vi "TestMode_Req_CMD_Abort.vi"(0 "Socket IP Address":string="192.168.1.100", 1 "Socket Port Number":u16=1600, 2 "Receipe Msg ID":i32=93, 3 "Receipe Message length":i32=36, 4 "Response ID":u8=94, 5 "error in (no error)":errorcluster, 6 "TestAmplitudeLoopC1":i32=500, 7 "TestFrequencyHigh":i32=500, 8 "TestAmplitudeLoopC2":i32=100, 9 "TestFrequencyLow":i32=450, 10 "TestPhaseLoopI":i32=300, 11 "TestAmplitude":i32=450, 12 "TestPhaseLoopCF":i32=500) -> (16 "Test Mode progress bar":string, 19 "error out":errorcluster)   [LabVIEW 2017]
panel:
  out "connection ID out":refnum<k5>
  # "Parameter Name                                        20KHz                                                                                                          \t40KHz\t\t\n\t                                        Default Value\t    Min Value\t       Max Value\t                                     Default Value         \tMin Value\t            Max Value\nTestAmplitudeLoopC1   100                         1                        20000                                               205                            1                             20000\nTestAmplitudeLoopC2   300                         1                        20000                                               370                            1                             20000\nTestPhaseLoopI               450                         50                      500                                                   60                             50                               500\nTestPhaseLoopCF           450                         50                       500                                                  200                           50                               500\nTestFrequencyHigh        20450                   Note                    Note                                                40900                      Note                           Note\nTestFrequencyLow          19450                   Note                   Note                                                38900                       Note                           Note\nTestAmplitude                 50                           10                       100                                                  50                             10                                100\n\nNote:  FreqLow and FreqHigh cannot cross and must remain within the band"
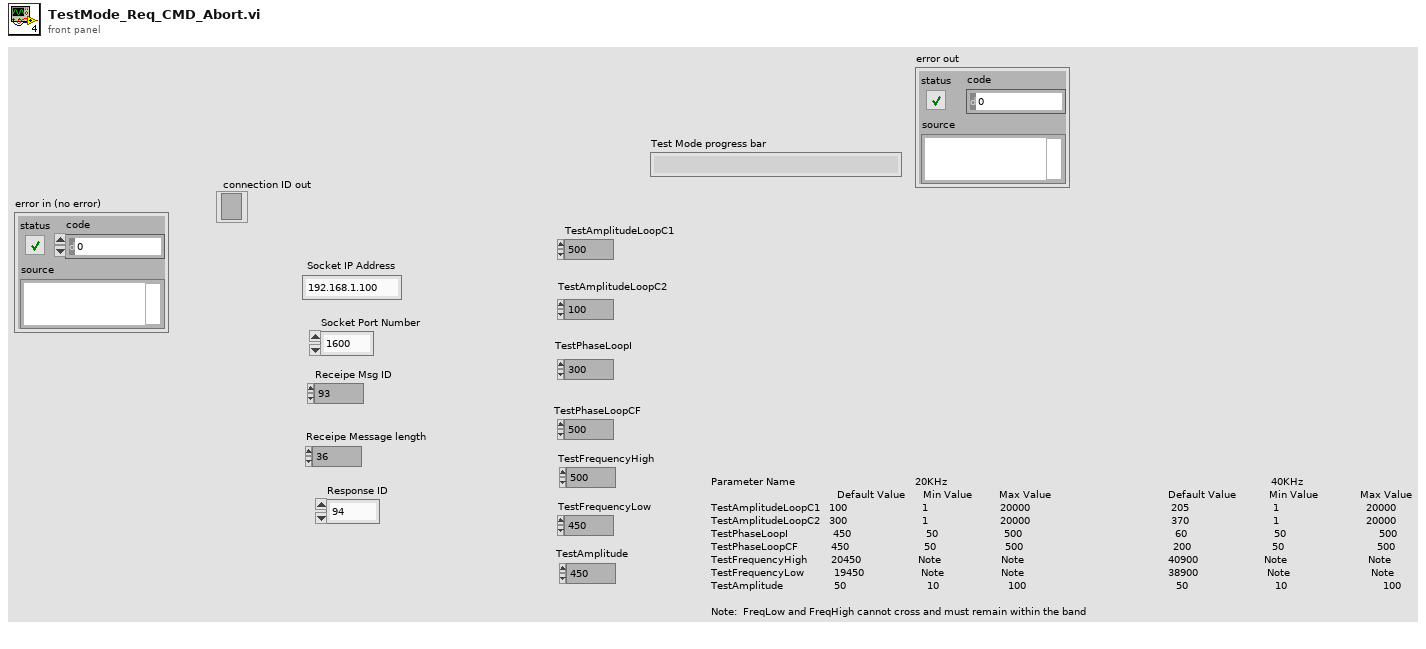
[diagram p1: front panel]
types:
  T1 = cluster{"Seek Request Message Length to DB ":i32, "Seek Request Message ID to DB":i32}
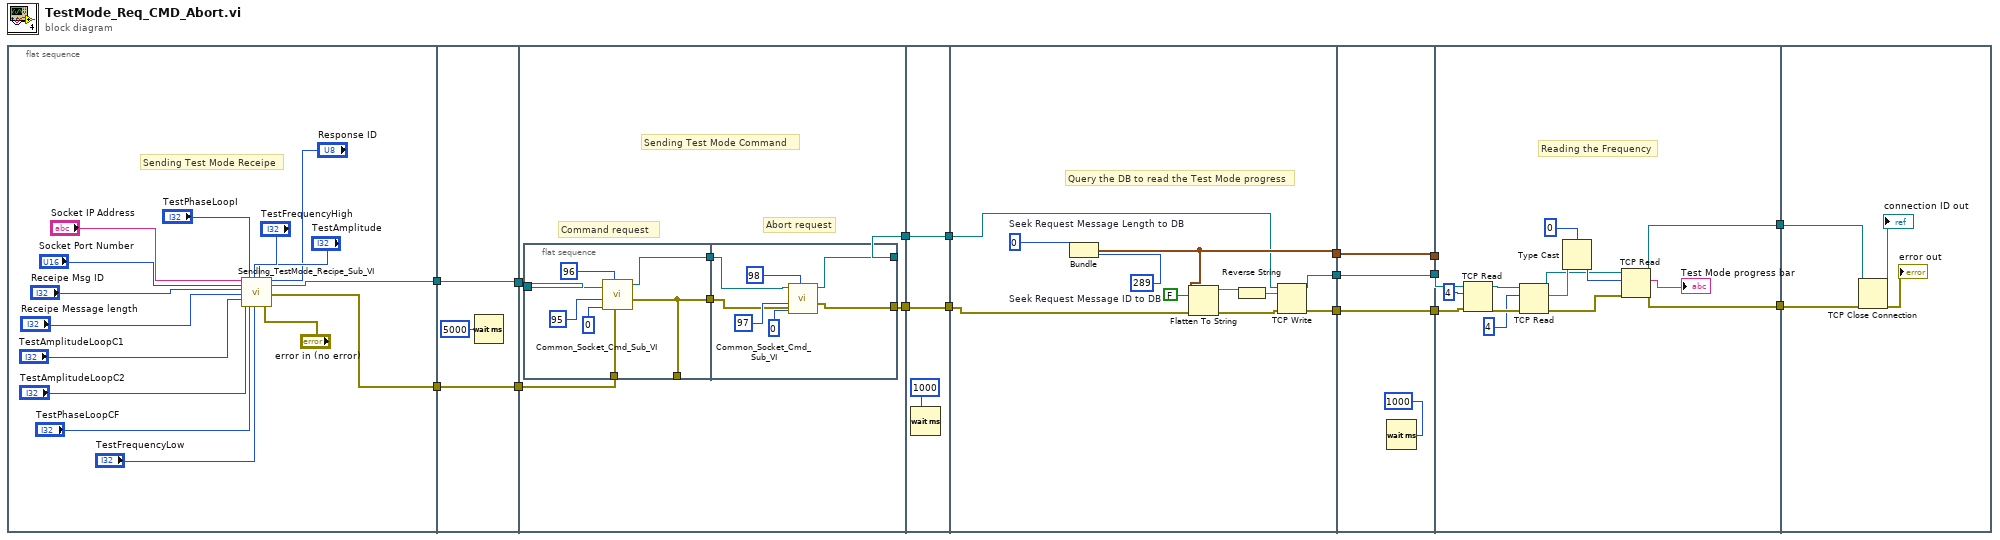
[diagram p0: block diagram]
diagram:
  n1 = flat-sequence {
    tunnel: [w31] -> w16
    tunnel: [w30] -> w15
    tunnel: w16 -> [w33]
    tunnel: w15 -> [w32]
    tunnel: [w33] -> w14
    tunnel: [w32] -> w13
    tunnel: w14 -> [w40]
    tunnel: w13 -> [w39]
    tunnel: [w35] -> w5
    tunnel: [w38] -> w3
    tunnel: w5 -> [w57]
    tunnel: [w57] -> w4
    tunnel: w3 -> [w56]
    tunnel: [w56] -> w2
    tunnel: w4 -> [w59]
    tunnel: w2 -> [w60]
    tunnel: [w62] -> w12
    tunnel: [w61] -> w11
    tunnel: [w58] -> w10
    tunnel: w12 -> [w72]
    tunnel: [w72] -> w9
    tunnel: w11 -> [w71]
    tunnel: [w71] -> w8
    tunnel: w10 -> [w70]
    tunnel: [w70] -> w7
    tunnel: w9 -> [_]
    tunnel: w8 -> [w85]
    tunnel: w7 -> [w84]
    tunnel: [w86] -> w6
    tunnel: [w73] -> w1
    tunnel: w6 -> [w88]
    tunnel: w1 -> [w87]
    frame #0 {
      # "Sending Test Mode Receipe"
      n2 = call "Sending_TestMode_Recipe_Sub_VI.vi"("Socket IP Address"="Socket IP Address", "Socket Port Numeber"="Socket Port Number", "Receipe Msg ID"="Receipe Msg ID", "Receipe Message length"="Receipe Message length", "TestAmplitudeLoopC1"="TestAmplitudeLoopC1", "TestAmplitudeLoopC2"="TestAmplitudeLoopC2", "TestPhaseLoopI"="TestPhaseLoopI", "TestPhaseLoopCF"="TestPhaseLoopCF", "TestFrequencyHigh"="TestFrequencyHigh", "TestFrequencyLow"="TestFrequencyLow", "TestAmplitude"="TestAmplitude", "error in (no error)"="error in (no error)", "Response ID"="Response ID") -> ("connection ID"=w31:refnum<k5>, "error out"=w30:errorcluster)  [unwired: 5 in]
    }
    frame #1 {
      n3 = Wait (ms)(milliseconds to wait=u32 5000) -> ()  [unwired: 1 out]
    }
    frame #2 {
      # "Abort request"
      # "Command request"
      # "Sending Test Mode Command"
      n4 = flat-sequence {
        tunnel: w40 -> [w47]
        tunnel: w39 -> [w46]
        tunnel: [w41] -> w37
        tunnel: [w45] -> w36
        tunnel: [w41] -> _
        tunnel: [w48] -> w38
        tunnel: w37 -> [w50]
        tunnel: w36 -> [w51]
        tunnel: [w49] -> w35
        frame #0 {
          n5 = call "Common_Socket_Cmd_Sub_VI.vi"("Common Socket Error in"=w46, "Response ID 1"=u8 96, "Operation Message Length 1"=0, "Operation Message ID 1"=95, "connection ID"=w47) -> ("error out"=w41:errorcluster, "connection ID"=w45:refnum<k5>)  [unwired: 4 in, 1 out]
        }
        frame #1 {
          n6 = call "Common_Socket_Cmd_Sub_VI.vi"("Common Socket Error in"=w50, "Response ID 1"=u8 98, "Operation Message Length 1"=0, "Operation Message ID 1"=97, "connection ID"=w51) -> ("error out"=w49:errorcluster, "connection ID"=w48:refnum<k5>)  [unwired: 4 in, 1 out]
        }
      }
    }
    frame #3 {
      n7 = Wait (ms)(milliseconds to wait=u32 1000) -> ()  [unwired: 1 out]
    }
    frame #4 {
      w63 = 289  # Seek Request Message ID to DB
      w64 = 0  # Seek Request Message Length to DB
      # "Query the DB to read the Test Mode progress"
      n8 = Bundle("Seek Request Message Length to DB"=w64, "Seek Request Message ID to DB"=w63) -> (w62:T1)  [unwired: 1 in]
      n9 = Flatten To String(anything=w62, prepend array or string size? (T)=FALSE, error in (no error)=w59) -> (data string=w68:string, error out=w66:errorcluster)  [unwired: 1 in, 1 out]
      n10 = Reverse String(1:w68) -> (0:w67:string)
      n11 = TCP Write(connection ID=w60, data in=w67, error in (no error)=w66) -> (connection ID out=w61:refnum<k5>, error out=w58:errorcluster)  [unwired: 1 in, 1 out]
    }
    frame #5 {
      n12 = Wait (ms)(milliseconds to wait=u32 1000) -> ()  [unwired: 1 out]
    }
    frame #6 {
      # "Reading the Frequency"
      n13 = TCP Read(connection ID=w85, bytes to read=4, error in (no error)=w84) -> (connection ID out=w82:refnum<k5>, error out=w81:errorcluster)  [unwired: 2 in, 1 out]
      n14 = TCP Read(connection ID=w82, bytes to read=4, error in (no error)=w81) -> (connection ID out=w76:refnum<k5>, data out=w79:string, error out=w75:errorcluster)  [unwired: 2 in]
      n15 = Type Cast(type=0 ("bytes to read"), x=w79) -> (*(type *) &x=w77:i32)
      n16 = TCP Read(connection ID=w76, bytes to read=w77, error in (no error)=w75) -> (connection ID out=w86:refnum<k5>, data out=→"Test Mode progress bar":string, error out=w73:errorcluster)  [unwired: 2 in]
    }
    frame #7 {
      n17 = TCP Close Connection(connection ID=w88, error in (no error)=w87) -> (connection ID out=→"connection ID out":refnum<k5>, error out=→"error out":errorcluster)  [unwired: 1 in]
    }
  }
